vi "RFSA 5668 Scanning Speed Benchmark IQ.vi"() -> ()   [LabVIEW 2017]
doc: "Demonstrates how to acquire a spectrum using the RF vector signal analyzer. This example shows how to configure NI-RFSA for spectrum acquisition, how to set the resolution bandwidth and reference level, and how to read power spectra while changing the center frequency in each iteration of the sweep while keeping the span constant. The spectrum is displayed on the graph. <B>Note</B> This example illustrates how to perform multiple spectrum acquisitions with different center frequency values. If you need to acquire a spectrum with a span wider than the instantaneous bandwidth of the device, use the Getting Started Spectrum example."
uses:
  <vilib>/Utility/error.llb/DialogType.ctl
  <vilib>/Analysis/1siggen.llb/Ramp Pattern by Delta.vi
  <instrlib>/niRFSA/niRFSA.llb/niRFSA Fetch IQ (Complex WDT 1Rec 1Chan).vi
  <vilib>/measure/maspectr.llb/FFT Power Spectrum and PSD for 1 Chan (CDB).vi
  <vilib>/Utility/file.llb/Write Delimited Spreadsheet (DBL).vi
  <vilib>/measure/NI_MAPro.lvlib
  <vilib>/Analysis/NI_AALBase.lvlib
panel:
  out "Ramp Pattern":dbl[](array[numeric]) format="%#_6p"
  in  "Spacing":dbl=1.0 format="%#_6p"
  in  "Start Carrier Frequency":dbl=1.0 format="%#_6p"
  in  "End Carrier Frequency":dbl=1.0 format="%#_6p"
  in  "Frequency Settling":dbl=1.0
  out "Waveform Graph 4":cluster{"f0":dbl, "df":dbl, "magnitude":dbl[]}(graph)
  out "Waveform Graph 3":cluster{"f0":dbl, "df":dbl, "magnitude":dbl[]}(graph)
  out "Waveform Graph 2":cluster{"f0":dbl, "df":dbl, "magnitude":dbl[]}(graph)
  out "Waveform Graph":cluster{"f0":dbl, "df":dbl, "magnitude":dbl[]}(graph)
  out "LO1 Frequencies":dbl[](array[numeric]) format="%#_6p"
  out "Samples per record":i64 format="%.0p"
  in  "Resolution Bandwidth (Hz)":dbl=10000.0 caption="Resolution Bandwidth" format="%#_6p"
  in  "stop":bool
  in  "Resource Name":refnum<k15>="RFSA"
  in  "Reference Level (dBm)":dbl format="%.2f"
  # "Overview: Demonstrates how to acquire a spectrum using the RF vector signal analyzer. \nRequirements: NI-RFSA\nInstructions:\n1. Change the Resource Name to your device.\n2. Run the VI.\n3. Click Stop to stop the VI."
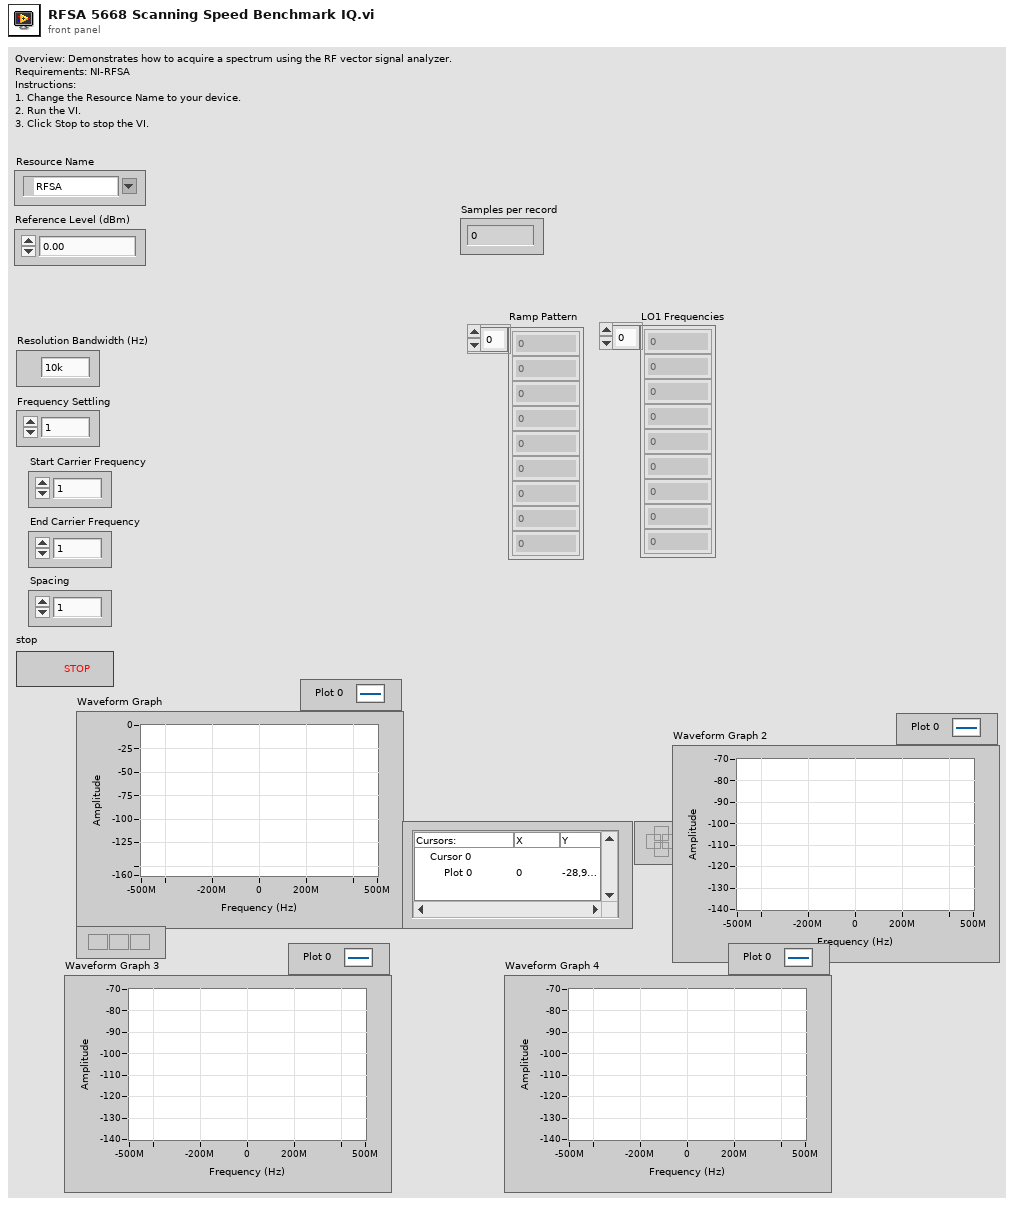
[diagram p1: front panel]
types:
  T1 = typedef "DialogType.ctl" = u16
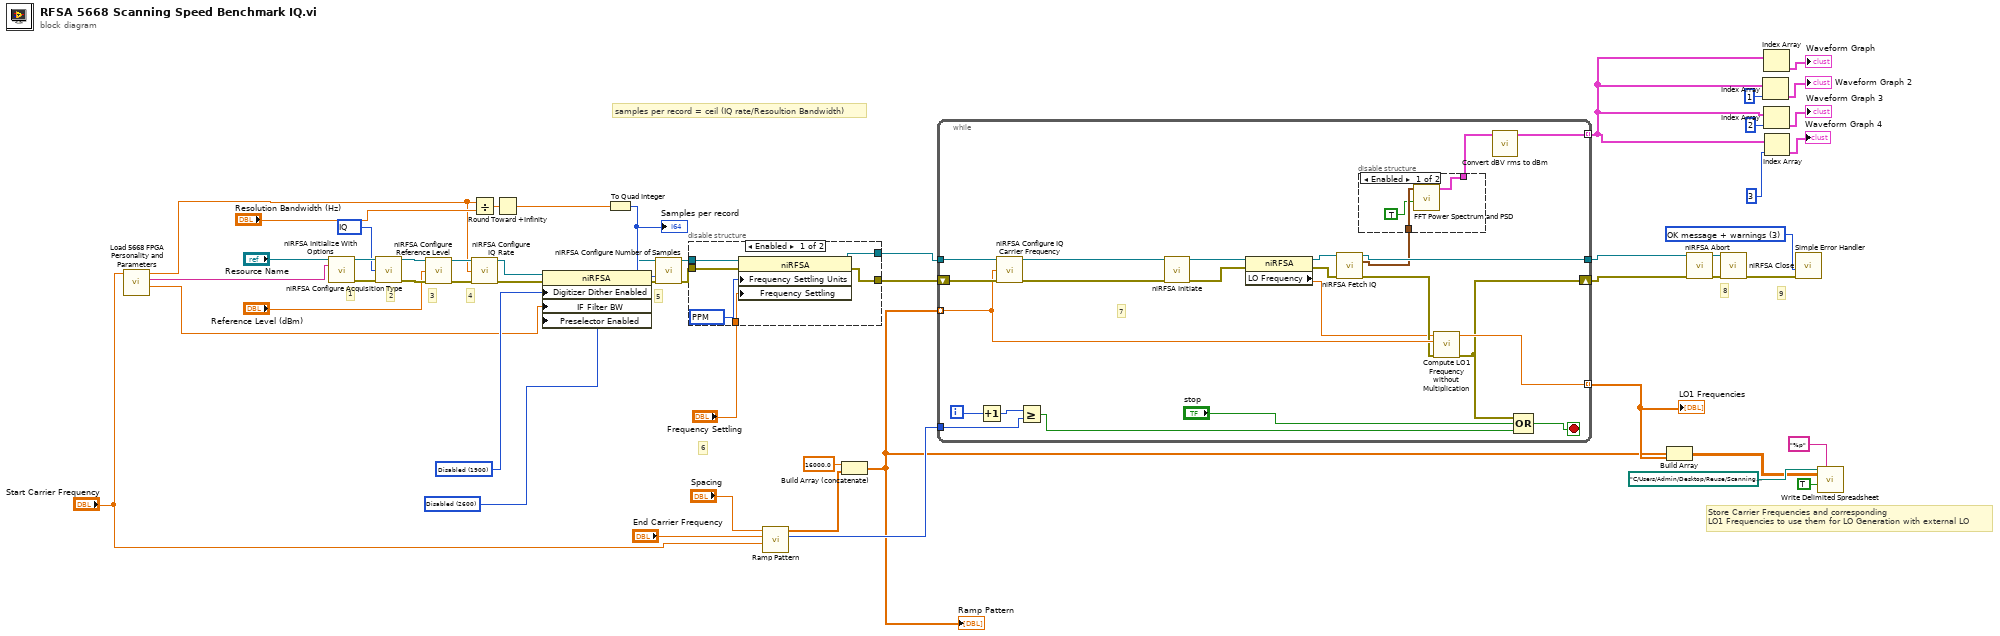
[diagram p0: block diagram]
diagram:
  w20 = 2600 items=["Disabled"=2600, "Enabled when in Signal Path"=2601, "Enabled"=2602] ("Signal Path:Advanced:Downconverter Preselector Enabled")
  w21 = 1900 items=["Disabled"=1900, "Enabled"=1901] ("Signal Path:Digitizer Dither Enabled")
  w49 = T1 3 items=["no dialog", "OK message", "continue or stop message", "OK message + warnings", "continue/stop + warnings"] ("type of dialog (OK msg:1)")
  w50 = 100 items=["IQ"=100, "Spectrum"=101] ("Acquisition:Acquisition Type")
  # "Store Carrier Frequencies and corresponding \nLO1 Frequencies to use them for LO Generation with external LO"
  # "samples per record = ceil (IQ rate/Resoultion Bandwidth)"
  # "8"
  # "9"
  # "6"
  # "5"
  # "4"
  # "3"
  # "2"
  # "1"
  n1 = call "Load 5668 FPGA Personality and Parameters.vi"("Start Carrier Frequency in"="Start Carrier Frequency") -> ("Signal Path:IF Filter Bandwidth"=w16:dbl, "option string"=w41:string, "IQ rate (S/s)"=w15:dbl)  [unwired: 8 in]
  n2 = call <instrlib>:"niRFSA Initialize With Options.vi"("resource name"="Resource Name", "option string"=w41) -> ("instrument handle out"=w53:refnum<k15>, "error out"=w52:errorcluster)  [unwired: 12 in]
  n3 = call <instrlib>:"niRFSA Configure Acquisition Type.vi"("instrument handle"=w53, "acquisition type"=w50, "error in"=w52) -> ("instrument handle out"=w46:refnum<k15>, "error out"=w45:errorcluster)  [unwired: 11 in]
  n4 = call <instrlib>:"niRFSA Configure Reference Level.vi"("instrument handle"=w46, "reference level (dBm)"="Reference Level (dBm)", "error in"=w45) -> ("instrument handle out"=w43:refnum<k15>, "error out"=w44:errorcluster)  [unwired: 11 in]
  n5 = Divide(x=w15, y="Resolution Bandwidth (Hz)") -> (x/y=w37:dbl)
  n6 = call <instrlib>:"niRFSA Configure IQ Rate.vi"("instrument handle"=w43, "IQ rate (S/s)"=w15, "error in"=w44) -> ("instrument handle out"=w23:refnum<k15>, "error out"=w29:errorcluster)  [unwired: 11 in]
  n7 = Round Toward +Infinity(x=w37) -> (ceil(x): smallest int >= x=w35:dbl)
  n8 = property class="niRFSA"(reference=w23, error in=w29, "Digitizer Dither Enabled"=w21, "IF Filter BW"=w16, "Preselector Enabled"=w20) -> (reference out=w22:refnum<k15>, error out=w24:errorcluster)
  n9 = To Quad Integer(1:w35) -> (0:w34:i64)
  "Samples per record" <- w34
  n10 = call <instrlib>:"niRFSA Configure Number of Samples.vi"("instrument handle"=w22, "samples per record"=w34, "error in"=w24) -> ("instrument handle out"=w39:refnum<k15>, "error out"=w38:errorcluster)  [unwired: 11 in]
  n11 = disable-structure shown="Enabled" {
    disable-tunnel: [w59 w60] -> w47
    disable-tunnel: [w58 w61] -> w40
    disable-tunnel: w39 -> [w56 w61]
    disable-tunnel: w38 -> [w55 w60]
    disable-tunnel: "Frequency Settling" -> [w54 _]
    frame Enabled {
      w57 = 2000 items=["PPM"=2000, "Seconds After Lock"=2001, "Seconds After I/O"=2002] ("Signal Path:Advanced:Frequency Settling Units")
      n12 = property class="niRFSA"(reference=w56, error in=w55, "Frequency Settling Units"=w57, "Frequency Settling"=w54) -> (reference out=w58:refnum<k15>, error out=w59:errorcluster)
    }
    frame Disabled {
    }
  }
  n13 = call-poly <vilib>:"Ramp Pattern.vi"("start"="Start Carrier Frequency", "end"="End Carrier Frequency", "delta"="Spacing") -> ("samples"=w17:i32, "Ramp Pattern"=w2:dbl[])  [unwired: 6 in, 1 out]
  n14 = Build Array (concatenate)(16000.0 ("element"), w2) -> (w1:dbl[])
  "Ramp Pattern" <- w1
  n15 = while {
    shift-right: [w65] -> w32
    shift-left: w47 -> [w84]
    tunnel: w40 -> [w83]
    tunnel: [w72] -> w33
    tunnel: [w67] -> w11 mode=indexing
    tunnel: w17 -> [w70]
    tunnel: w1 -> [w68] mode=indexing
    tunnel: [w63] -> w5 mode=indexing
    i -> [w78]
    stop <- w80 stop-if-true
    # "7"
    n16 = Increment(x=w78) -> (x+1=w77:i32)
    n17 = call <instrlib>:"niRFSA Configure IQ Carrier Frequency.vi"("instrument handle"=w83, "carrier frequency"=w68, "error in"=w84) -> ("instrument handle out"=w82:refnum<k15>, "error out"=w81:errorcluster)  [unwired: 11 in]
    n18 = Greater Or Equal?(x=w77, y=w70) -> (x >= y?=w69:bool)
    n19 = call <instrlib>:"niRFSA Initiate.vi"("instrument handle"=w82, "error in"=w81) -> ("instrument handle out"=w75:refnum<k15>, "error out"=w76:errorcluster)  [unwired: 12 in]
    n20 = property class="niRFSA"(reference=w75, error in=w76) -> (reference out=w73:refnum<k15>, error out=w74:errorcluster, "LO Frequency"=w62:dbl)
    n21 = call-poly <instrlib>:"niRFSA Fetch IQ.vi"("instrument handle"=w73, "error in"=w74) -> ("instrument handle out"=w72:refnum<k15>, "data"=w71:waveform(cdb), "error out"=w66:errorcluster)  [unwired: 11 in]
    n22 = disable-structure shown="Enabled" {
      disable-tunnel: w71 -> [w87 _]
      disable-tunnel: [w85 _] -> w64
      frame Enabled {
        n23 = call-poly <vilib>:"FFT Power Spectrum and PSD.vi"("dB On (F)"=TRUE, "time signal"=w87) -> ("Power Spectrum / PSD"=w85:cluster{"f0":dbl, "df":dbl, "magnitude":dbl[]})  [unwired: 6 in, 3 out]
      }
      frame Disabled {
      }
    }
    n24 = call "Compute LO1 Frequency without Multiplication.vi"("error in (no error)"=w66, "Carrier Frequency"=w68, "Input LO1 Frequency"=w62) -> ("error out"=w65:errorcluster, "Output LO1 Frequency"=w67:dbl)  [unwired: 7 in]
    n25 = call "Convert dBV rms to dBm.vi"("Power Spectrum / PSD (dBV rms)"=w64) -> ("Power Spectrum / PSD (dBm)"=w63:cluster{"f0":dbl, "df":dbl, "magnitude":dbl[]})  [unwired: 9 in, 1 out]
    n26 = Compound Arithmetic op=OR(w65, "stop", w69) -> (w80:bool)
  }
  "LO1 Frequencies" <- w11
  n27 = Build Array(w1, w11) -> (w10:dbl[][])
  n28 = call <instrlib>:"niRFSA Abort.vi"("instrument handle"=w33, "error in"=w32) -> ("instrument handle out"=w31:refnum<k15>, "error out"=w30:errorcluster)  [unwired: 12 in]
  n29 = call <instrlib>:"niRFSA Close.vi"("instrument handle"=w31, "error in"=w30) -> ("error out"=w51:errorcluster)  [unwired: 13 in]
  n30 = Index Array(array=w5, index=1) -> (element=→"Waveform Graph 2":cluster{"f0":dbl, "df":dbl, "magnitude":dbl[]})
  n31 = Index Array(array=w5) -> (element=→"Waveform Graph":cluster{"f0":dbl, "df":dbl, "magnitude":dbl[]})  [unwired: 1 in]
  n32 = Index Array(array=w5, index=2) -> (element=→"Waveform Graph 3":cluster{"f0":dbl, "df":dbl, "magnitude":dbl[]})
  n33 = Index Array(array=w5, index=3) -> (element=→"Waveform Graph 4":cluster{"f0":dbl, "df":dbl, "magnitude":dbl[]})
  n34 = call <vilib>:"Simple Error Handler.vi"("type of dialog (OK msg:1)"=w49, "error in (no error)"=w51) -> ()  [unwired: 3 in, 5 out]
  n35 = call-poly <vilib>:"Write Delimited Spreadsheet.vi"("file path (dialog if empty)"=path "C:/Users/Admin/Desktop/Reuse/Scanning Speed PXIe 5668/LO1 Frequencies.txt", "format (%.3f)"="%p", "2D data"=w10, "append to file? (new file:F)"=TRUE) -> ()  [unwired: 10 in, 2 out]
